vi "Sig_AO_Create.vi"(0 "reference in":refnum<class "Sig_AO.lvclass">, 5 "error in (no error)":errorcluster) -> (14 "reference out":refnum<class "Sig_AO.lvclass">, 19 "error out":errorcluster)   [LabVIEW 2019, in "Sig_AO.lvclass"]
doc: "Constructor."
uses:
  Sig_AO.lvclass
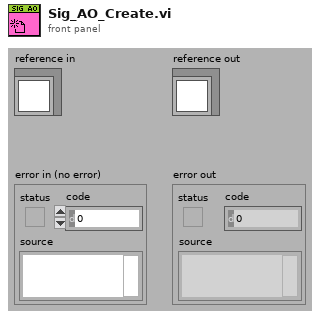
[diagram p1: front panel]
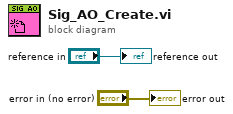
[diagram p0: block diagram]
diagram:
  "error out" <- "error in (no error)"
  "reference out" <- "reference in"
